vi "Get Comparison Value.vi"(8 "error in (no error)":errorcluster, 11 "Test in":refnum<class "Test.lvclass">) -> (0 "error out":errorcluster, 1 "Invert Result":bool, 2 "Data String":string)   [LabVIEW 2018, in "Test.lvclass"]
doc: "Pulls the comparison value (as a string, still has to be converted for other data types) and the invert status from the JSON config"
uses:
  Test.lvclass
  cead256c-5a43-4736-851c-7a506df39983.vi
  Test Class String IDs.vi
  <vilib>/JDP Science/JSONtext/JSON text to Variant.vi
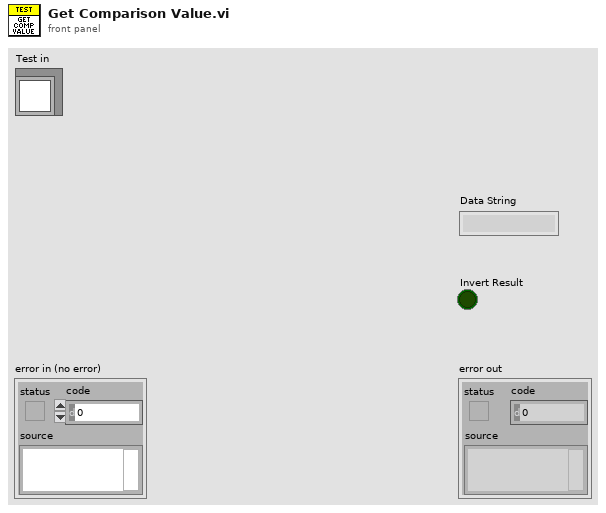
[diagram p1: front panel]
types:
  T1 = cluster{"Comparison Value 1":string, "Comparison Value 2":string, "Invert Result":string, "Assert VI Name":string, "Data Type":string, "Builder User Name":string, "Build Timestamp":string, "Failure Action":string, "Comment":string, "Assert Name":string, "Description":string, "Evaluation String":string}
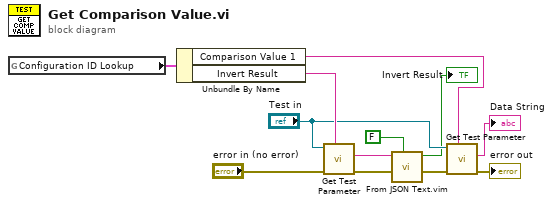
[diagram p0: block diagram]
diagram:
  n1 = global read "Test Class String IDs.vi" "Configuration ID Lookup"() -> (w11:T1)
  n2 = Unbundle By Name(w11) -> ("Comparison Value 1"=w9:string, "Invert Result"=w10:string)
  n3 = call "Get Test Parameter.vi"("Data Value ID"=w10, "error in (no error)"="error in (no error)", "Test in"="Test in") -> ("error out"=w12:errorcluster, "Test Parameter"=w7:string)  [unwired: 6 in, 1 out]
  n4 = call "From JSON Text.vim"("Data Type and Default Value"=FALSE, "error in (no error)"=w12, "JSON"=w7) -> ("error out"=w8:errorcluster, "Data out"=→"Invert Result":bool)  [unwired: 7 in]
  n5 = call "Get Test Parameter.vi"("Data Value ID"=w9, "error in (no error)"=w8, "Test in"="Test in") -> ("error out"=→"error out":errorcluster, "Test Parameter"=→"Data String":string)  [unwired: 6 in, 1 out]
